vi "Create.vi"(8 "error in (no error)":errorcluster, 10 "ID tag":string, 11 "Instrument in":refnum<class>) -> (0 "error out":errorcluster, 3 "Instrument Pointer":refnum<class "InstrPtr.lvclass">, 5 "Type Specifier":refnum<class>)   [LabVIEW 2017, in "InstrPtr.lvclass"]
doc: "Create a new InstrPtr and place this object on the heap.\n\nSet an \"ID tag\" if you create more than one instance of the same object class.\n\nIt is recommended to bundle the resultant InstrPtr with its Type Specifier. That way, you can feed the bundle to Dereference later on."
uses:
  InstrPtr.lvclass
  InstrPtr.lvclass/InstrPtr.ctl
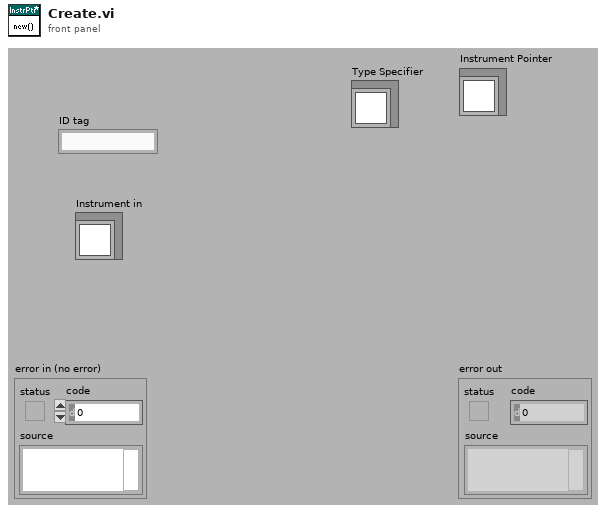
[diagram p1: front panel]
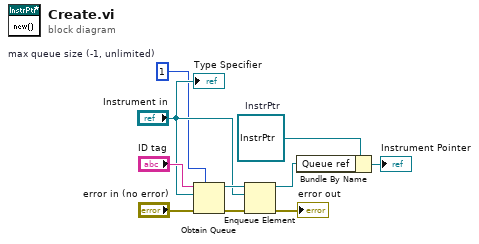
[diagram p0: block diagram]
diagram:
  w1 = 1  # max queue size (-1, unlimited)
  w8 = refnum<class "InstrPtr.lvclass"> refnum  # InstrPtr
  n1 = Obtain Queue(max queue size (-1, unlimited)=w1, name (unnamed)="ID tag", element data type="Instrument in", error in (no error)="error in (no error)") -> (queue out=w7:refnum<queue>, error out=w2:errorcluster)  [unwired: 1 in, 1 out]
  n2 = Enqueue Element(queue=w7, element="Instrument in", error in (no error)=w2) -> (queue out=w6:refnum<queue>, error out=→"error out":errorcluster)  [unwired: 2 out]
  n3 = Bundle By Name(cluster=w8, "Queue ref"=w6) -> (→"Instrument Pointer":refnum<class "InstrPtr.lvclass">)
  "Type Specifier" <- "Instrument in"
